vi "Set Sweep Time.vi"(7 "Sweep Time Param (sweep time)":T1, 8 "error in (no error)":errorcluster, 9 "time":dbl[unit], 10 "Channel (0: Channel 1)":T2 items=["Channel 1", "Channel 2"], 11 "VISA resource name":refnum<visa-resource-name>) -> (0 "error out":errorcluster, 3 "VISA resource name out":refnum<visa-resource-name>)   [LabVIEW 2009, in "Tektronix AFG 3000 Series.lvlib"]
doc: "Sets the sweep time, hold time (htime), or return time (rtime) of a Tektronix AFG 3000 series function generator. The sweep time does not include hold time and return time, and return time does not include hold time. <B>Note:</B> will coerce the time to the acceptable range (1 ms - 300 s for sweep time, and 0-300 s for the other two)."
uses:
  Tektronix AFG 3000 Series.lvlib
  controls.llb/Channel.ctl
  controls.llb/Sweep Time Parameter.ctl
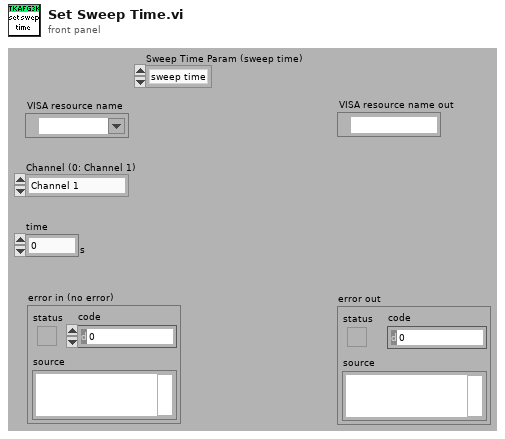
[diagram p1: front panel]
types:
  T1 = typedef "Sweep Time Parameter.ctl" = enum16{"sweep time", "hold time", "return time"}
  T2 = typedef "Channel.ctl" = u16
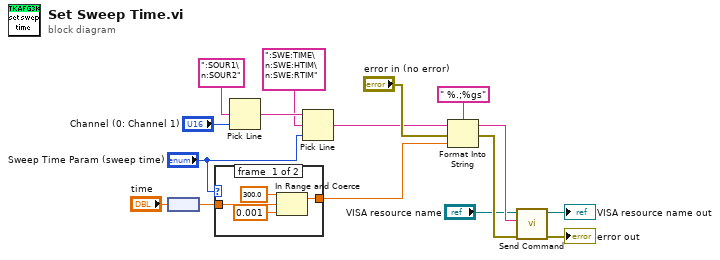
[diagram p0: block diagram]
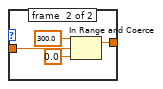
[diagram p2: hidden frame]
diagram:
  n1 = node("time") -> (w9:dbl)
  n2 = case shown="Default" "Sweep Time Param (sweep time)" {
    tunnel: w9 -> [w20 w24]
    tunnel: [w17 w21] -> w8
    frame #0 {
      n3 = In Range and Coerce(upper limit=300.0, x=w20, lower limit=0.001) -> (coerced(x)=w17:dbl)  [unwired: 1 out]
    }
    frame #1 {
      n4 = In Range and Coerce(upper limit=300.0, x=w24, lower limit=0.0) -> (coerced(x)=w21:dbl)  [unwired: 1 out]
    }
  }
  n5 = Pick Line(multi-line string=":SOUR1\n:SOUR2", line index="Channel (0: Channel 1)") -> (output string=w7:string)  [unwired: 1 out]
  n6 = Pick Line(string ("")=w7, multi-line string=":SWE:TIME\n:SWE:HTIM\n:SWE:RTIM", line index="Sweep Time Param (sweep time)") -> (output string=w4:string)
  n7 = Format Into String(format string=" %.;%gs", initial string=w4, error in="error in (no error)", w8) -> (resulting string=w13:string, error out=w11:errorcluster)
  n8 = call "Send Command.vi"("error in (no error)"=w11, "write buffer"=w13, "VISA resource name"="VISA resource name") -> ("error out"=→"error out":errorcluster, "VISA resource name out"=→"VISA resource name out":refnum<visa-resource-name>)  [unwired: 7 out]
